vi "Tracking with Motor BACKUP.vi"() -> ()   [LabVIEW 2011]
panel:
  out "Actual Goal\nPosition":dbl(knob) scale=-1.0..1.0
  out "Current\nPosition":dbl(knob) scale=-1.0..1.0
  in  "Right of Goal":dbl(slide) scale=-1.0..1.0
  in  "Right Limit hit?":bool
  in  "Left Limit hit?":bool
  out "Updated Position":T1(array[cluster])
  in  "Motor Speed":dbl
  in  "stop":bool
  out "Fire!":bool
  in  "Target Info":T1(array[cluster])
  in  "Left of Goal":dbl(slide) scale=-1.0..1.0
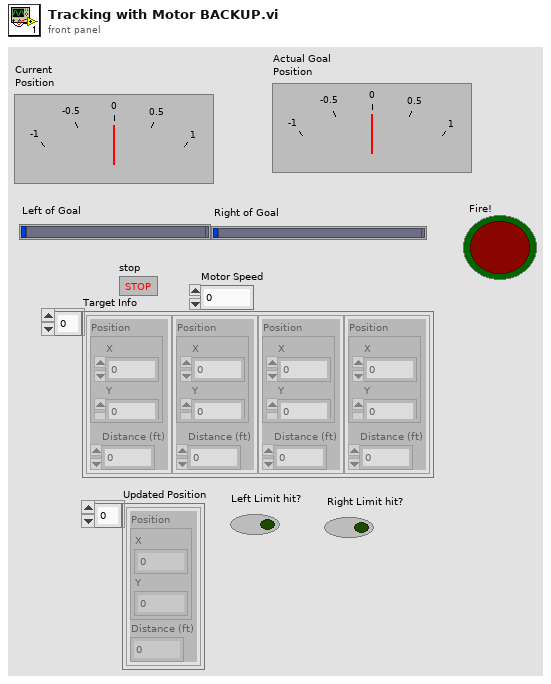
[diagram p1: front panel]
types:
  T1 = cluster{"Position":cluster{"X":dbl, "Y":dbl}, "Distance (ft)":dbl}[]
  T2 = cluster{"Target Info[0]":cluster{"Position":cluster{"X":dbl, "Y":dbl}, "Distance (ft)":dbl}, "Target Info[1]":cluster{"Position":cluster{"X":dbl, "Y":dbl}, "Distance (ft)":dbl}, "Target Info[2]":cluster{"Position":cluster{"X":dbl, "Y":dbl}, "Distance (ft)":dbl}, "Target Info[3]":cluster{"Position":cluster{"X":dbl, "Y":dbl}, "Distance (ft)":dbl}, "Target Info[4]":cluster{"Position":cluster{"X":dbl, "Y":dbl}, "Distance (ft)":dbl}, "Target Info[5]":cluster{"Position":cluster{"X":dbl, "Y":dbl}, "Distance (ft)":dbl}, "Target Info[6]":cluster{"Position":cluster{"X":dbl, "Y":dbl}, "Distance (ft)":dbl}, "Target Info[7]":cluster{"Position":cluster{"X":dbl, "Y":dbl}, "Distance (ft)":dbl}, "Target Info[8]":cluster{"Position":cluster{"X":dbl, "Y":dbl}, "Distance (ft)":dbl}}
  T3 = cluster{"Position":cluster{"X":dbl, "Y":dbl}, "Distance (ft)":dbl}
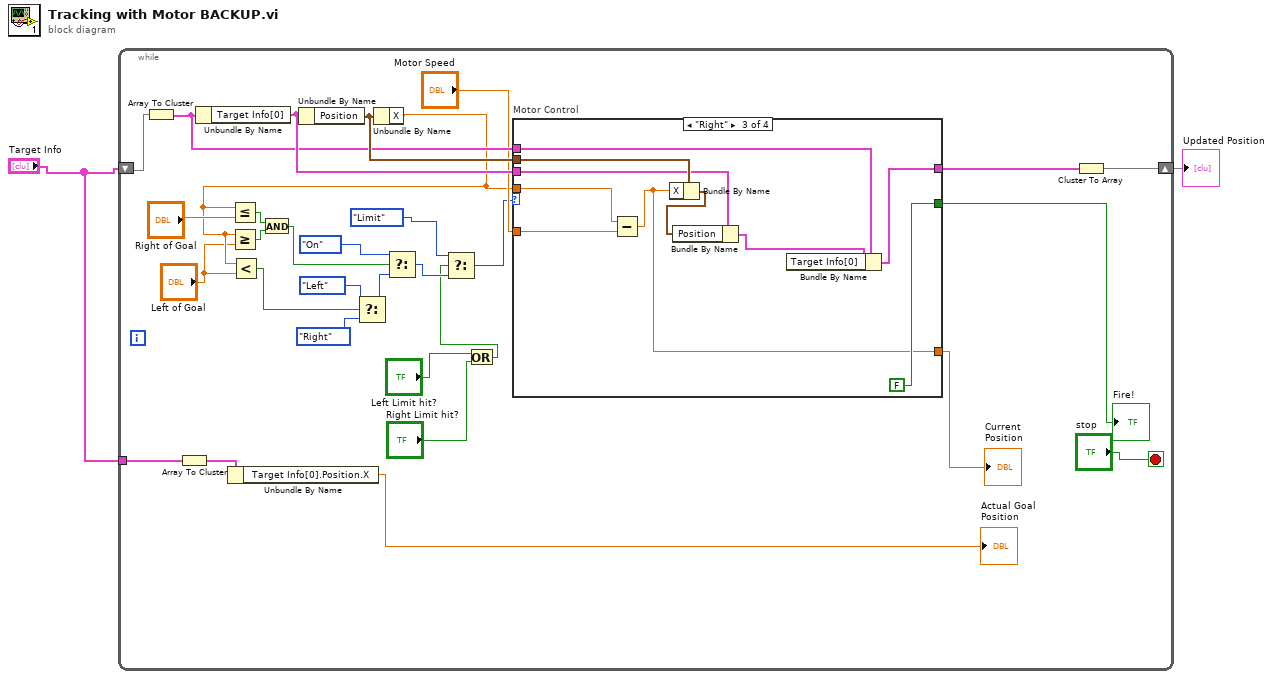
[diagram p0: block diagram]
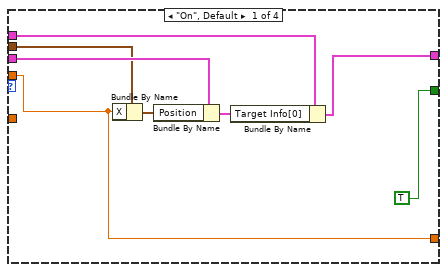
[diagram p2: hidden frame]
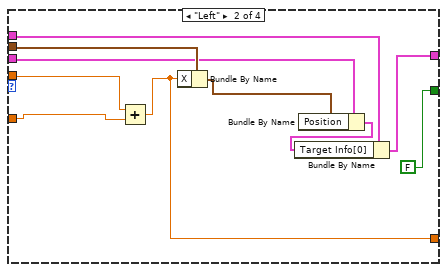
[diagram p3: hidden frame]
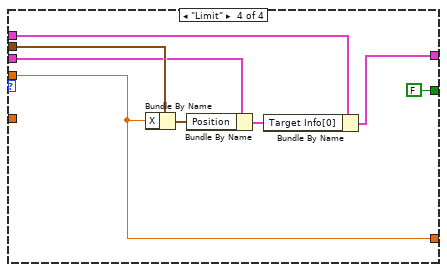
[diagram p4: hidden frame]
diagram:
  n1 = while {
    shift-right: [w26] -> w2
    shift-left: "Target Info" -> [w28]
    tunnel: "Target Info" -> [w6]
    stop <- "stop" stop-if-true
    n2 = Array To Cluster(array=w28) -> (cluster=w23:T2)
    n3 = Array To Cluster(array=w6) -> (cluster=w5:T2)
    n4 = Unbundle By Name(w23) -> ("Target Info[0]"=w24:T3)
    n5 = Unbundle By Name(w5) -> ("Target Info[0].Position.X"=→"Actual Goal\nPosition":dbl)
    n6 = Unbundle By Name(w24) -> ("Position"=w25:cluster{"X":dbl, "Y":dbl})
    n7 = Unbundle By Name(w25) -> ("X"=w9:dbl)
    n8 = Less Or Equal?(x=w9, y="Right of Goal") -> (x <= y?=w12:bool)
    n9 = Greater Or Equal?(x=w9, y="Left of Goal") -> (x >= y?=w11:bool)
    n10 = Less?(x=w9, y="Left of Goal") -> (x < y?=w7:bool)
    n11 = And(x=w12, y=w11) -> (x .and. y?=w10:bool)
    n12 = Select(t=enum16{"On", "Left", "Right", "Limit"}."Left", s=w7, f=enum16{"On", "Left", "Right", "Limit"}."Right") -> (s? t:f=w32:enum16{"On", "Left", "Right", "Limit"})
    n13 = Select(t=enum16{"On", "Left", "Right", "Limit"}."On", s=w10, f=w32) -> (s? t:f=w21:enum16{"On", "Left", "Right", "Limit"})
    n14 = Or(x="Left Limit hit?", y="Right Limit hit?") -> (x .or. y?=w17:bool)
    n15 = Select(t=enum16{"On", "Left", "Right", "Limit"}."Limit", s=w17, f=w21) -> (s? t:f=w20:enum16{"On", "Left", "Right", "Limit"})
    n16 = case "Motor Control" shown="\"Right\"" w20 {
      tunnel: [TRUE FALSE FALSE FALSE] -> w30
      tunnel: w9 -> [w33 w44 w59 w61]
      tunnel: [w36 w43 w56 w65] -> w27
      tunnel: w25 -> [w34 w46 w55 w63]
      tunnel: w24 -> [w35 w45 w54 w62]
      tunnel: w23 -> [w37 w47 w53 w64]
      tunnel: "Motor Speed" -> [_ w42 w52 _]
      tunnel: [w33 w41 w51 w61] -> w4
      frame "On", Default {
        n17 = Bundle By Name(cluster=w34, "X"=w33) -> (w38:cluster{"X":dbl, "Y":dbl})
        n18 = Bundle By Name(cluster=w35, "Position"=w38) -> (w39:T3)
        n19 = Bundle By Name(cluster=w37, "Target Info[0]"=w39) -> (w36:T2)
      }
      frame "Left" {
        n20 = Add(x=w44, y=w42) -> (x+y=w41:dbl)
        n21 = Bundle By Name(cluster=w46, "X"=w41) -> (w48:cluster{"X":dbl, "Y":dbl})
        n22 = Bundle By Name(cluster=w45, "Position"=w48) -> (w49:T3)
        n23 = Bundle By Name(cluster=w47, "Target Info[0]"=w49) -> (w43:T2)
      }
      frame "Right" {
        n24 = Subtract(x=w59, y=w52) -> (x-y=w51:dbl)
        n25 = Bundle By Name(cluster=w55, "X"=w51) -> (w58:cluster{"X":dbl, "Y":dbl})
        n26 = Bundle By Name(cluster=w54, "Position"=w58) -> (w57:T3)
        n27 = Bundle By Name(cluster=w53, "Target Info[0]"=w57) -> (w56:T2)
      }
      frame "Limit" {
        n28 = Bundle By Name(cluster=w63, "X"=w61) -> (w66:cluster{"X":dbl, "Y":dbl})
        n29 = Bundle By Name(cluster=w62, "Position"=w66) -> (w67:T3)
        n30 = Bundle By Name(cluster=w64, "Target Info[0]"=w67) -> (w65:T2)
      }
    }
    "Fire!" <- w30
    "Current\nPosition" <- w4
    n31 = Cluster To Array(cluster=w27) -> (array=w26:T1)
  }
  "Updated Position" <- w2
